vi "RobotDriveOpen6MotorWithVenom.vi"(0 "Left Motor 1":u8=255, 1 "Left Motor 2":u8=255, 2 "Left Motor 3":u8=255, 3 "Right Motor 1":u8=255, 4 "Right Motor 2":u8=255, 5 "Right Motor 3":u8=255, 7 "error in (no error)":errorcluster, 8 "Left Motor 1 Inverted":bool, 9 "Right Motor 1 Inverted":bool, 10 "Left Motor 2 Inverted":bool, 11 "Right Motor 2 Inverted":bool, 12 "Left Motor 3 Inverted":bool, 13 "Right Motor 3 Inverted":bool) -> (20 "RobotDriveDevRef":T1={"DevStatus"={"status"=FALSE, "code"=0, "source"=""}, "Motors[]"=[], "Square Inputs"=FALSE, "Max Output"=1.0}, 27 "error out":errorcluster)   [LabVIEW 2019, in "ArgosLib.lvlib"]
doc: "Opens a reference to the robot drive for a two-, four-, or six-motor robot using Talon SR motor controllers connected via CAN bus.\n\nFor 2-motor drive, connect Left Motor 1 and Right Motor 1.\nFor 4-motor drive, connect Left Motor 2 and Right Motor 2 in addition to the 2-motor drive connections.\nFor 6-motor drive, connect Left Motor 3 and Right Motor 3 in addition to the 4-motor drive connections.\n\nInversions are optional and are set to false if disconnected.\n\nThis software is licensed. Open the labview\\readme\\WPI Robotics Library Open Source License.txt file for more information."
uses:
  ArgosLib.lvlib
  <vilib>/Rock Robotics/WPI/RobotDrive/WPI_RobotDriveDevRef.ctl
  <vilib>/Rock Robotics/WPI/MotorControl/WPI_MotorControlDeviceRef.ctl
  <vilib>/Rock Robotics/WPI/MotorControl/WPI_MotorControlType.ctl
  <vilib>/Rock Robotics/SystemInterfaces/DIO/FPGA_DIOPWMChannel.ctl
  <vilib>/Rock Robotics/WPI/PWM/WPI_PWMDeadband.ctl
  <vilib>/Rock Robotics/SystemInterfaces/DIO/FPGA_DIOChannel.ctl
  <vilib>/Rock Robotics/WPI/SafetyOutput/WPI_SafetyOutputConfigMenu.ctl
  <vilib>/Playing With Fusion Inc/Playing With Fusion Lib for FRC/PWF_Venom_LabVIEW/PwF_Venom.lvlib
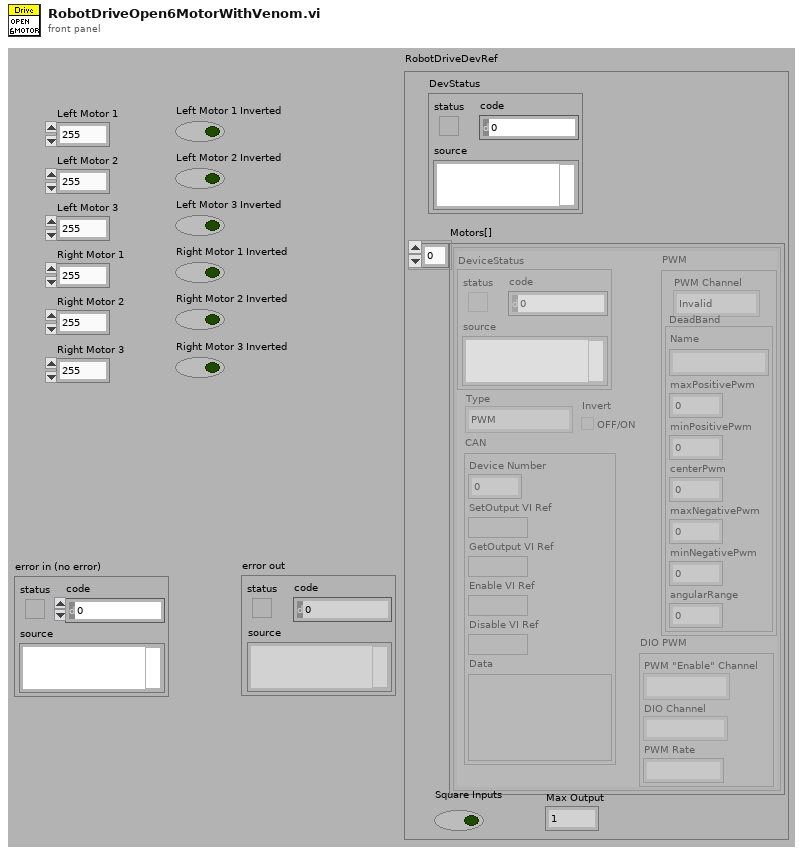
[diagram p1: front panel]
types:
  T1 = typedef "WPI_RobotDriveDevRef.ctl" = cluster{"DevStatus":errorcluster, "Motors[]":T2[], "Square Inputs":bool, "Max Output":dbl}
  T2 = typedef "WPI_MotorControlDeviceRef.ctl" = cluster{"DeviceStatus":errorcluster, "Type":T3, "PWM":cluster{"PWM Channel":T4, "DeadBand":T5}, "CAN":cluster{"Device Number":u8, "SetOutput VI Ref":variant, "GetOutput VI Ref":variant, "Enable VI Ref":variant, "Disable VI Ref":variant, "Data":variant}, "Invert":bool, "DIO PWM":cluster{"PWM \"Enable\" Channel":T4, "DIOChannel":T6, "PWM Rate":dbl}}
  T3 = typedef "WPI_MotorControlType.ctl" = enum16{"PWM", "CAN", "DIO PWM"}
  T4 = typedef "FPGA_DIOPWMChannel.ctl" = enum8{"PWM 0", "PWM 1", "PWM 2", "PWM 3", "PWM 4", "PWM 5", "PWM 6", "PWM 7", "PWM 8", "PWM 9", "PWM MXP 0", "PWM MXP 1", "PWM MXP 2", "PWM MXP 3", "PWM MXP 4", "PWM MXP 5", "PWM MXP 6", "PWM MXP 7", "PWM MXP 8", "PWM MXP 9", "Invalid"}
  T5 = typedef "WPI_PWMDeadband.ctl" = cluster{"Name":string, "maxPositivePwm":i32, "minPositivePwm":i32, "centerPwm":i32, "maxNegativePwm":i32, "minNegativePwm":i32, "angularRange":u16}
  T6 = typedef "FPGA_DIOChannel.ctl" = enum8{"DIO 0", "DIO 1", "DIO 2", "DIO 3", "DIO 4", "DIO 5", "DIO 6", "DIO 7", "DIO 8", "DIO 9", "DIO MXP 0", "DIO MXP 1", "DIO MXP 2", "DIO MXP 3", "DIO MXP 4", "DIO MXP 5", "DIO MXP 6", "DIO MXP 7", "DIO MXP 8", "DIO MXP 9", "DIO MXP 10", "DIO MXP 11", "DIO MXP 12", "DIO MXP 13", "DIO MXP 14", "DIO MXP 15", "SPI Port CS1", "SPI Port CS2", "SPI Port CS3", "SPI Port MISO", "SPI Port MOSI", "Invalid"}
  T7 = typedef "WPI_SafetyOutputConfigMenu.ctl" = enum16{"Enable", "Disable"}
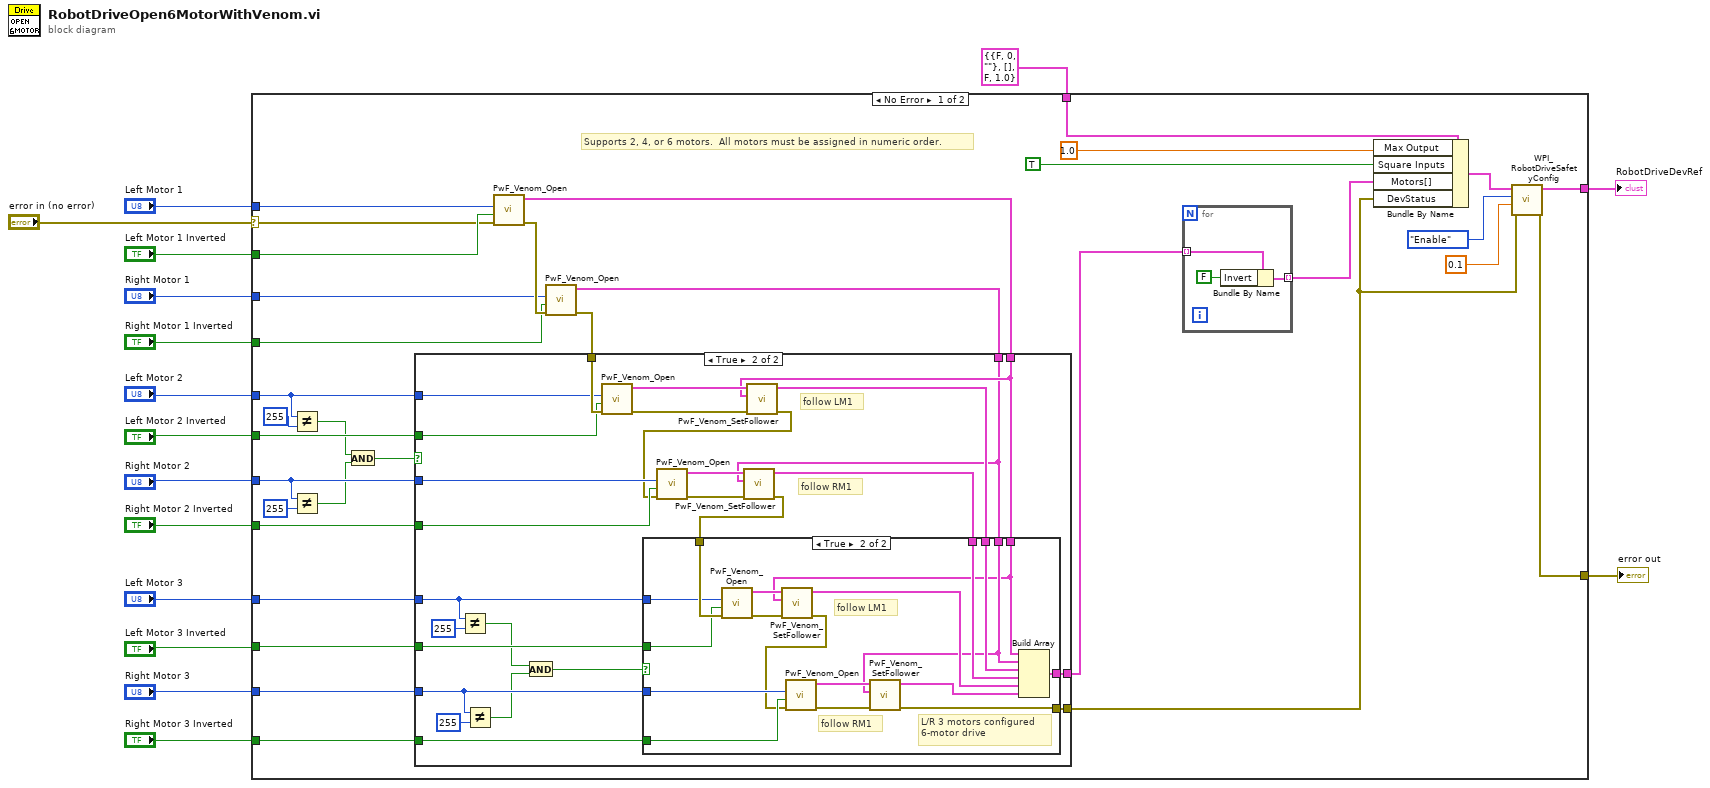
[diagram p0: block diagram]
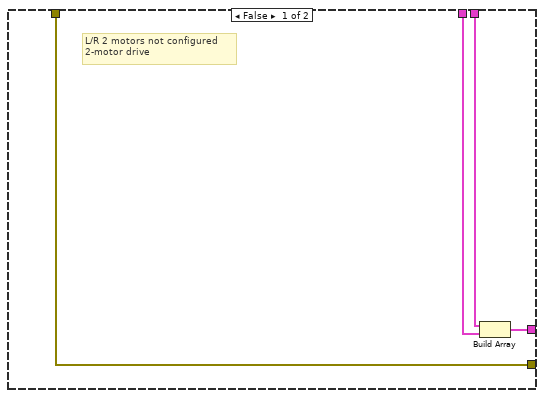
[diagram p2: hidden frame]
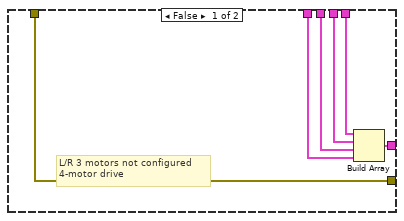
[diagram p3: hidden frame]
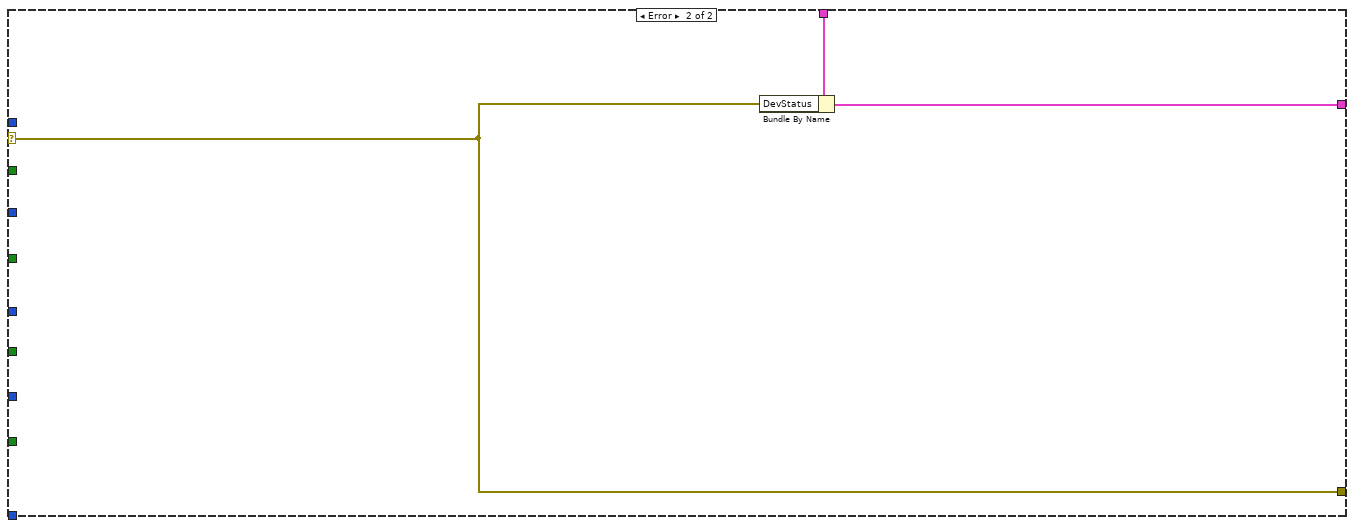
[diagram p4: hidden frame]
diagram:
  n1 = case shown="No Error" "error in (no error)" {
    selector: "error in (no error)" -> [w28 w107]
    tunnel: [w38 w108] -> w16
    tunnel: T1 {"DevStatus"={"status"=FALSE, "code"=0, "source"=""}, "Motors[]"=[], "Square Inputs"=FALSE, "Max Output"=1.0} ("RobotDriveDevRef") -> [w49 w109]
    tunnel: "Left Motor 1 Inverted" -> [w45 _]
    tunnel: "Right Motor 1 Inverted" -> [w44 _]
    tunnel: "Right Motor 2 Inverted" -> [w42 _]
    tunnel: "Left Motor 2 Inverted" -> [w43 _]
    tunnel: [w39 w107] -> w9
    tunnel: "Left Motor 3 Inverted" -> [w35 _]
    tunnel: "Right Motor 3 Inverted" -> [w34 _]
    tunnel: "Left Motor 1" -> [w32 _]
    tunnel: "Right Motor 1" -> [w31 _]
    tunnel: "Left Motor 2" -> [w27 _]
    tunnel: "Right Motor 2" -> [w24 _]
    tunnel: "Left Motor 3" -> [w30 _]
    tunnel: "Right Motor 3" -> [w29 _]
    frame No Error {
      # "Supports 2, 4, or 6 motors.  All motors must be assigned in numeric order."
      n2 = Not Equal?(x=w27, y=u8 255) -> (x != y?=w23:bool)
      n3 = Not Equal?(x=w24, y=u8 255) -> (x != y?=w22:bool)
      n4 = And(x=w23, y=w22) -> (x .and. y?=w21:bool)
      n5 = call <vilib>:"PwF_Venom_Open.vi"("error in"=w28, "Invert"=w45, "Device Number"=w32) -> ("error out"=w46:errorcluster, "Venom Ref"=w19:T2)  [unwired: 7 in]
      n6 = call <vilib>:"PwF_Venom_Open.vi"("error in"=w46, "Invert"=w44, "Device Number"=w31) -> ("error out"=w47:errorcluster, "Venom Ref"=w20:T2)  [unwired: 7 in]
      n7 = case shown="True" w21 {
        tunnel: w47 -> [w56 w82]
        tunnel: w43 -> [_ w81]
        tunnel: w42 -> [_ w80]
        tunnel: w35 -> [_ w79]
        tunnel: w34 -> [_ w78]
        tunnel: [w56 w77] -> w33
        tunnel: w30 -> [_ w71]
        tunnel: w29 -> [_ w72]
        tunnel: w27 -> [_ w76]
        tunnel: w24 -> [_ w75]
        tunnel: [w55 w67] -> w18
        tunnel: w19 -> [w54 w62]
        tunnel: w20 -> [w53 w57]
        frame False {
          # "L/R 2 motors not configured\n2-motor drive"
          n8 = Build Array(w54, w53) -> (w55:T2[])
        }
        frame True {
          # "follow LM1"
          # "follow RM1"
          n9 = Not Equal?(x=w71, y=u8 255) -> (x != y?=w69:bool)
          n10 = Not Equal?(x=w72, y=u8 255) -> (x != y?=w68:bool)
          n11 = And(x=w69, y=w68) -> (x .and. y?=w70:bool)
          n12 = call <vilib>:"PwF_Venom_Open.vi"("error in"=w82, "Invert"=w81, "Device Number"=w76) -> ("error out"=w64:errorcluster, "Venom Ref"=w66:T2)  [unwired: 7 in]
          n13 = call <vilib>:"PwF_Venom_SetFollower.vi"("error in"=w64, "LeaderDevRef"=w62, "PwFVenomDevRefIn"=w66) -> ("error out"=w63:errorcluster, "PwFVenomDevRefOut"=w65:T2)  [unwired: 7 in]
          n14 = call <vilib>:"PwF_Venom_Open.vi"("error in"=w63, "Invert"=w80, "Device Number"=w75) -> ("error out"=w59:errorcluster, "Venom Ref"=w61:T2)  [unwired: 7 in]
          n15 = call <vilib>:"PwF_Venom_SetFollower.vi"("error in"=w59, "LeaderDevRef"=w57, "PwFVenomDevRefIn"=w61) -> ("error out"=w58:errorcluster, "PwFVenomDevRefOut"=w60:T2)  [unwired: 7 in]
          n16 = case shown="True" w70 {
            tunnel: w58 -> [w88 w106]
            tunnel: w79 -> [_ w105]
            tunnel: w78 -> [_ w104]
            tunnel: [w88 w90] -> w77
            tunnel: w71 -> [_ w103]
            tunnel: w72 -> [_ w102]
            tunnel: [w87 w101] -> w67
            tunnel: w62 -> [w86 w89]
            tunnel: w57 -> [w85 w92]
            tunnel: w65 -> [w84 w100]
            tunnel: w60 -> [w83 w99]
            frame False {
              # "L/R 3 motors not configured\n4-motor drive"
              n17 = Build Array(w86, w85, w84, w83) -> (w87:T2[])
            }
            frame True {
              # "follow LM1"
              # "follow RM1"
              # "L/R 3 motors configured\n6-motor drive"
              n18 = call <vilib>:"PwF_Venom_Open.vi"("error in"=w106, "Invert"=w105, "Device Number"=w103) -> ("error out"=w96:errorcluster, "Venom Ref"=w98:T2)  [unwired: 7 in]
              n19 = call <vilib>:"PwF_Venom_SetFollower.vi"("error in"=w96, "LeaderDevRef"=w89, "PwFVenomDevRefIn"=w98) -> ("error out"=w95:errorcluster, "PwFVenomDevRefOut"=w97:T2)  [unwired: 7 in]
              n20 = call <vilib>:"PwF_Venom_Open.vi"("error in"=w95, "Invert"=w104, "Device Number"=w102) -> ("error out"=w91:errorcluster, "Venom Ref"=w94:T2)  [unwired: 7 in]
              n21 = call <vilib>:"PwF_Venom_SetFollower.vi"("error in"=w91, "LeaderDevRef"=w92, "PwFVenomDevRefIn"=w94) -> ("error out"=w90:errorcluster, "PwFVenomDevRefOut"=w93:T2)  [unwired: 7 in]
              n22 = Build Array(w89, w92, w100, w99, w97, w93) -> (w101:T2[])
            }
          }
        }
      }
      n23 = for {
        tunnel: w18 -> [w52] mode=indexing
        tunnel: [w50] -> w17 mode=indexing
        n24 = Bundle By Name(cluster=w52, "Invert"=FALSE) -> (w50:T2)
      }
      n25 = Bundle By Name(cluster=w49, "Max Output"=1.0, "Square Inputs"=TRUE ("DestroyPWM?"), "Motors[]"=w17, "DevStatus"=w33) -> (w40:T1)
      n26 = call <vilib>:"WPI_RobotDriveSafetyConfig.vi"("error in (no error)"=w33, "timeout (s)"=0.1, "mode"=WPI_SafetyOutputConfigMenu."Enable", "RobotDriveDevRef"=w40) -> ("error out"=w39:errorcluster, "RobotDriveDevRef"=w38:T1)  [unwired: 6 out]
    }
    frame Error {
      n27 = Bundle By Name(cluster=w109, "DevStatus"=w107) -> (w108:T1)
    }
  }
  "RobotDriveDevRef" <- w16
  "error out" <- w9
